vi "exit logic.vi"(0 "system state in":T1, 11 "exit":bool) -> (4 "system state out":T1, 15 "exit program":bool)   [LabVIEW 2016]
doc: "This subvi terminates the program no matter in what mode the program is.\n\nAlexis Lopez\nP350\nCSUSB Physics"
uses:
  typedefs/system state cluster.ctl
  typedefs/state enum.ctl
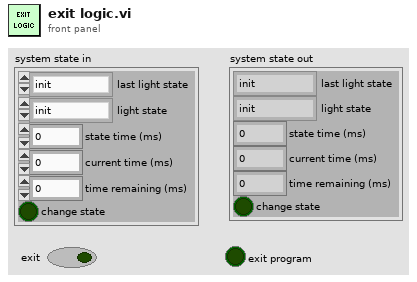
[diagram p1: front panel]
types:
  T1 = typedef "system state cluster.ctl" = cluster{"last light state":T2, "light state":T2, "state time (ms)":i32, "current time (ms)":i32, "time remaining (ms)":i32, "change state":bool}
  T2 = typedef "state enum.ctl" = enum16{"init", "idle", "left turn E", "go EW", "caution EW", "left turn W", "left turn N", "go NS", "caution NS", "left turn S", "blink on", "blink off", "all on test", "exit"}
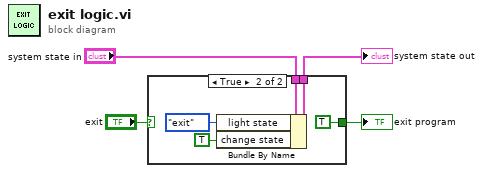
[diagram p0: block diagram]
diagram:
  n1 = case shown="True" "exit" {
    tunnel: [w5 w9] -> w4
    tunnel: "system state in" -> [w5 w10]
    tunnel: [_ TRUE] -> w2
    frame False {
    }
    frame True {
      n2 = Bundle By Name(cluster=w10, "light state"=state_enum."exit" ("current light state"), "change state"=TRUE) -> (w9:T1)
    }
  }
  "system state out" <- w4
  "exit program" <- w2
